vi "OpenG-INI Test Marshall-Unmarshall.vi"() -> ()   [LabVIEW 2019]
uses:
  OpenG-INI Test Cluster.ctl
  source/Serializer.openg-ini.lvclass
  C:/Program Files (x86)/National Instruments/LabVIEW 2019/vi.lib/LabVIEW Open Source Project/OpenSerializer/Serializer/Serializer.lvclass
  source/Serializer.openg-ini.lvclass/Serializer.openg-ini.ctl
  source/Write Floating Number Format.vi
  source/Read All Found_.vi
  source/Read Any Found_.vi
  <vilib>/LabVIEW Open Source Project/OpenSerializer/Serializer/Serializer.lvclass
panel:
  out "Any Found?":bool
  out "All Found?":bool
  in  "Floating Number Format":string="%.;%#_16g"
  out "error out":errorcluster
  out "Pass?":bool
  out "Data Cluster out":T1={"Top-Level Cluster"={"Boolean"=FALSE, "String"="", "Path"=path "", "Numeric"=0.0, "Enum"=enum."Item0", "Array"=[], "Sub-Cluster"={"Numeric"=4.0, "Boolean"=FALSE, "String"=""}}} {"Top-Level Cluster"."Numeric" format="%#_10g"}
  out "INI String":string
  in  "Data Cluster in":T1={"Top-Level Cluster"={"Boolean"=FALSE, "String"="Another test string", "Path"=path "C:/Windows", "Numeric"=3.141592654, "Enum"=enum."Item0", "Array"=[0.0, 1.0, 2.0, 3.0, 4.0, 5.0, 6.0], "Sub-Cluster"={"Numeric"=4.0, "Boolean"=TRUE, "String"="Test String Here"}}} {"Top-Level Cluster"."Numeric" format="%#_10g"}
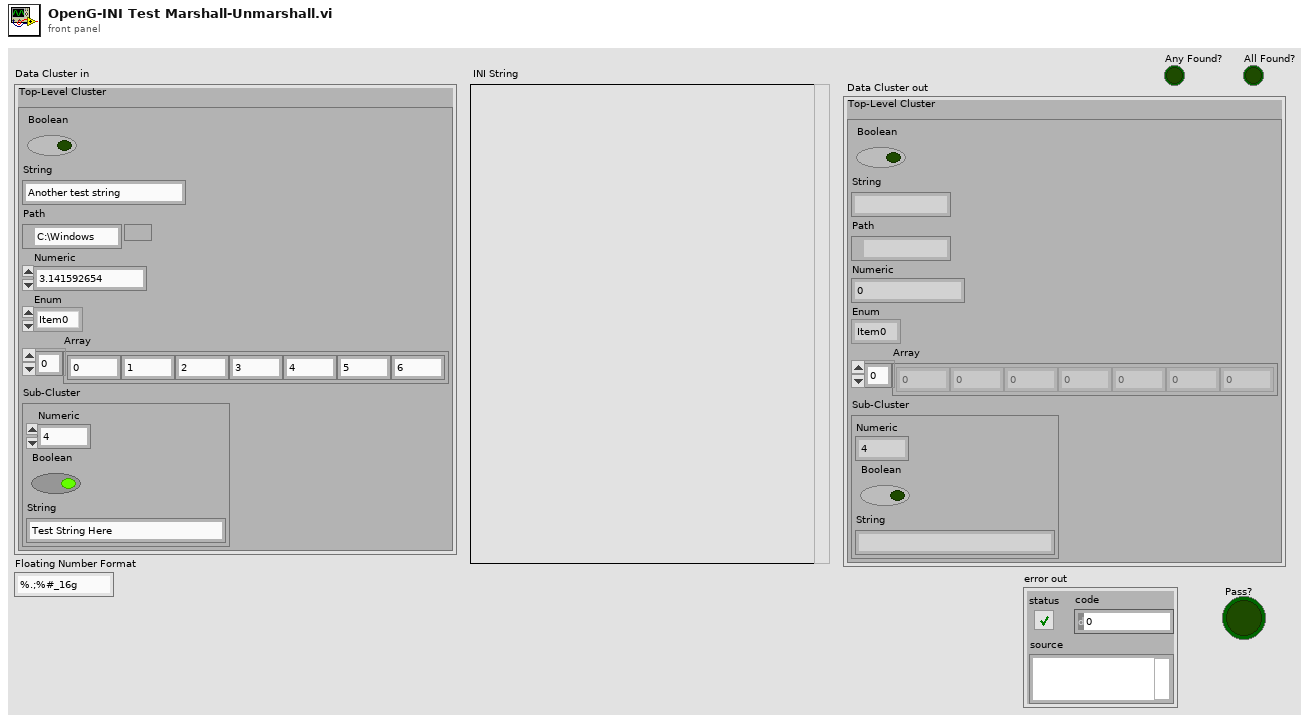
[diagram p1: front panel]
types:
  T1 = typedef "OpenG-INI Test Cluster.ctl" = cluster{"Top-Level Cluster":cluster{"Boolean":bool, "String":string, "Path":path, "Numeric":dbl, "Enum":enum16{"Item0", "Item1"}, "Array":dbl[], "Sub-Cluster":cluster{"Numeric":dbl, "Boolean":bool, "String":string}}}
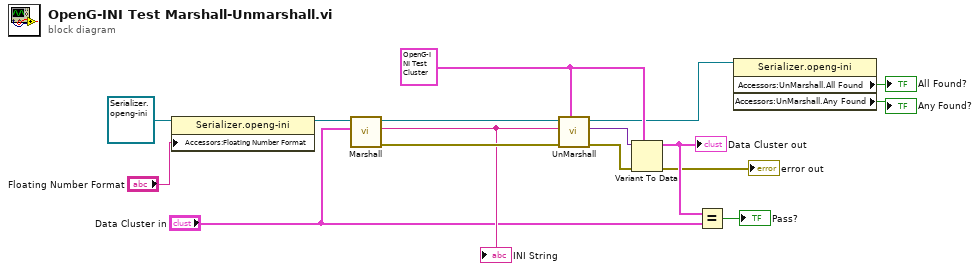
[diagram p0: block diagram]
diagram:
  w11 = T1 {"Top-Level Cluster"={"Boolean"=FALSE, "String"="", "Path"=path "", "Numeric"=0.0, "Enum"=enum."Item0", "Array"=[], "Sub-Cluster"={"Numeric"=4.0, "Boolean"=FALSE, "String"=""}}} ("Cluster")
  n1 = property class="Serializer.openg-ini"(reference=refnum<class "Serializer.openg-ini.lvclass"> refnum ("OpenSerializer.OpenG-ini.lvlib:Serializer.openg-ini"), "Accessors:Floating Number Format"="Floating Number Format") -> (reference out=w4:refnum<class "Serializer.openg-ini.lvclass">)  [unwired: 1 in, 1 out]
  n2 = call <vilib>:"Marshall.vi"("Variant"="Data Cluster in", "Serializer in"=w4) -> ("error out"=w16:errorcluster, "String"=w14:string, "Serializer out"=w15:refnum<class "Serializer.openg-ini.lvclass">)  [unwired: 7 in]
  "INI String" <- w14
  n3 = call <vilib>:"UnMarshall.vi"("Type"=w11, "error in (no error)"=w16, "String"=w14, "Serializer in"=w15) -> ("error out"=w13:errorcluster, "Variant"=w12:variant, "Serializer out"=w3:refnum<class "Serializer.openg-ini.lvclass">)  [unwired: 5 in]
  n4 = Variant To Data(error in=w13, type=w11, Variant=w12) -> (data=w10:T1, error out=→"error out":errorcluster)
  "Data Cluster out" <- w10
  n5 = Equal?(x=w10, y="Data Cluster in") -> (x = y?=→"Pass?":bool)
  n6 = property class="Serializer.openg-ini"(reference=w3) -> ("Accessors:UnMarshall.All Found"=→"All Found?":bool, "Accessors:UnMarshall.Any Found"=→"Any Found?":bool)  [unwired: 1 in, 2 out]
